vi "Import Export - Configuration Dialog.vi"(8 "error in":errorcluster, 11 "Item Ref in":T1 format="%.0x") -> (0 "error out":errorcluster, 3 "Item Ref out":T1 format="%.0x")   [LabVIEW 2017, in "PXImc System Explorer.lvlib"]
doc: "Goal of this VI is to prompt user to enter path t the configuration file and set Import or Export action over selected file.\n------------------------------------------------------------------------------------------------------\nIMPLEMENTATION\nCustom .net dialog window"
uses:
  PXImc System Explorer.lvlib
  <vilib>/NI Veristand/Custom Device API/Custom Device Item Ref.ctl
  <vilib>/event_ctls.llb/eventvkey.ctl
  Shared/Constants.vi
  <vilib>/NI Veristand/Custom Device API/Get Item Property (Path).vi
  <vilib>/NI Veristand/Custom Device API/Set Item Property (Path).vi
  <vilib>/NI VeriStand/Custom Device API/Custom Device API.lvlib
  Shared/PXImc Shared.lvlib
panel:
  in  "Forced?":bool=TRUE caption="Forced Import?"
  in  "dummy error cover":string
  in  "Import":bool
  in  "Close":bool
  in  "Export":bool
  in  "Configuration File Path":path
  # "File for Import/Export not found! Please seclect valid file to unlock this feature."
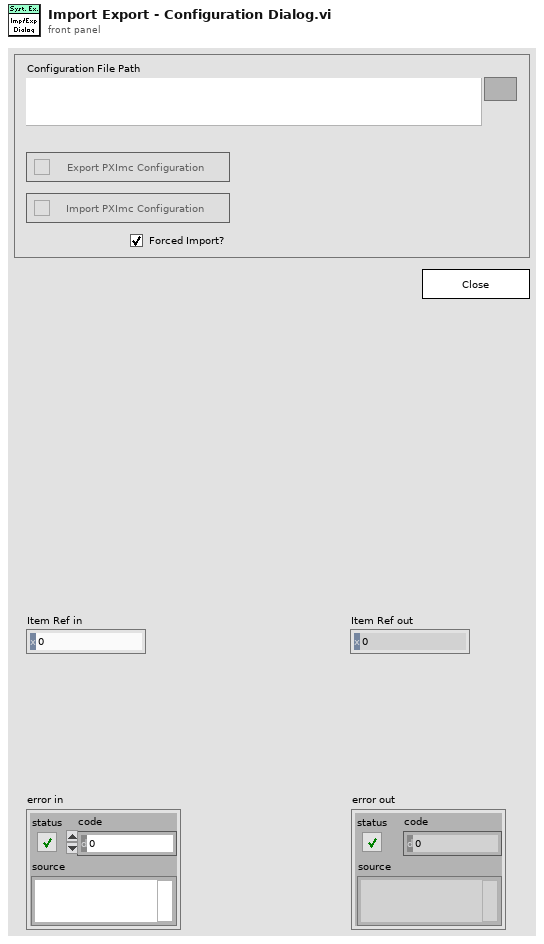
[diagram p1: front panel]
types:
  T1 = typedef "Custom Device API.lvlib/Custom Device Item Ref.ctl" = u64
  T2 = enum8{"Enabled", "Disabled", "Disabled and Grayed Out"}
  T3 = typedef "eventvkey.ctl" = enum16{"ASCII", "Enter", "Return", "Shift", "Ctrl", "Alt", "Cmd", "Opt", "Caps", "NumLock", "Clear", "Break", "Up", "Down", "Left", "Right", "Insert", "Delete", "Home", "End", "PageUp", "PageDown", "Escape", "Help", "Pause", "ScrollLock", "F1", "F2", "F3", "F4", "F5", "F6", "F7", "F8", "F9", "F10", "F11", "F12", "F13", "F14", "F15", "F16", "F17", "F18", "F19", "F20", "F21", "F22", "F23", "F24", "Play", "VolumeUp", "VolumeDown", "Mute", "Two Byte Char"}
  T4 = enum16{"open", "replace", "create", "open or create", "replace or create", "replace or create with confirmation"}
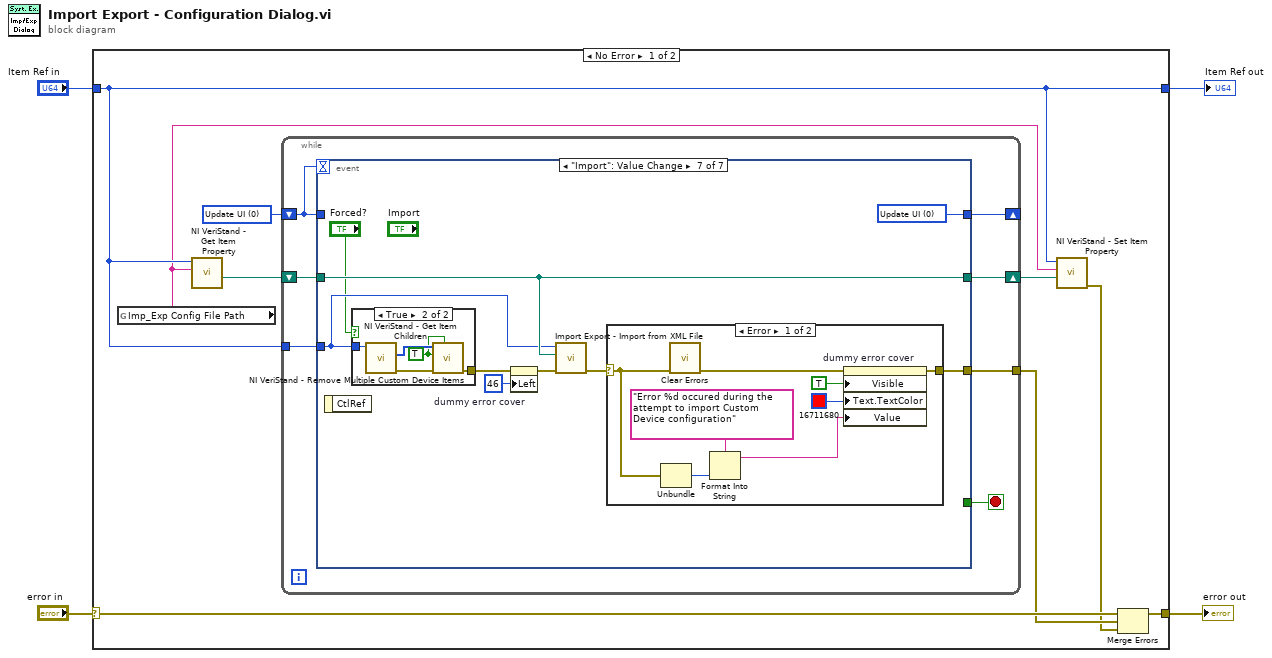
[diagram p0: block diagram]
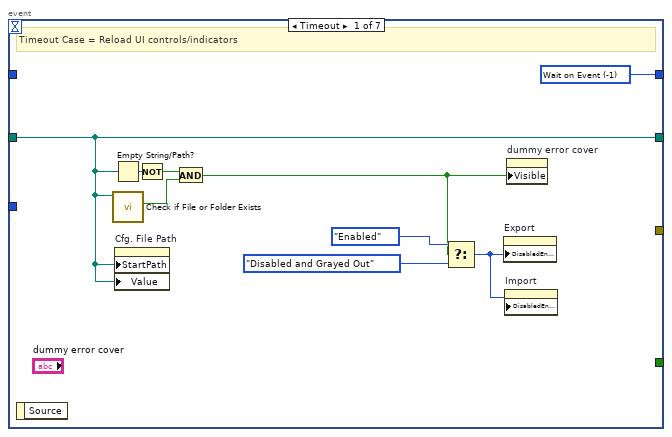
[diagram p2: hidden frame]
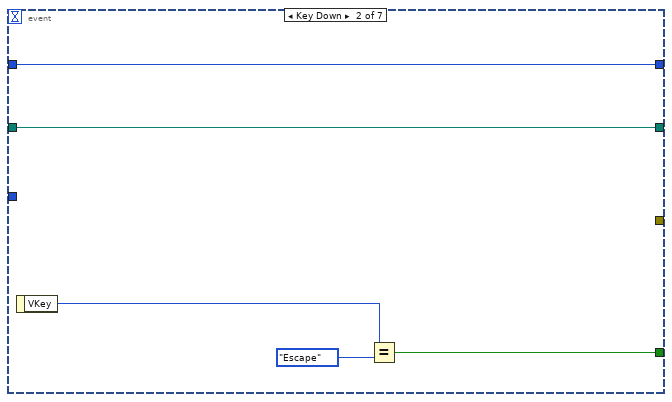
[diagram p3: hidden frame]
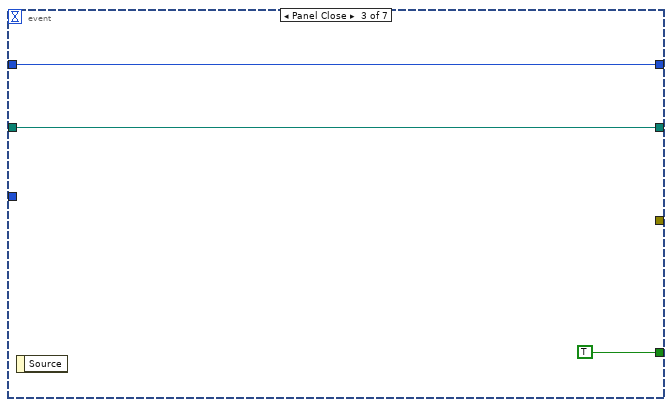
[diagram p4: hidden frame]
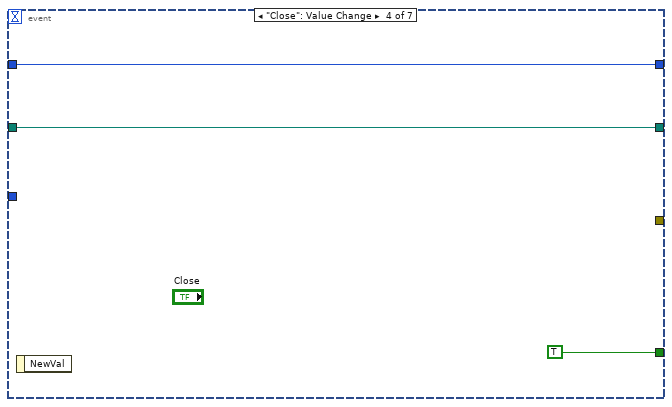
[diagram p5: hidden frame]
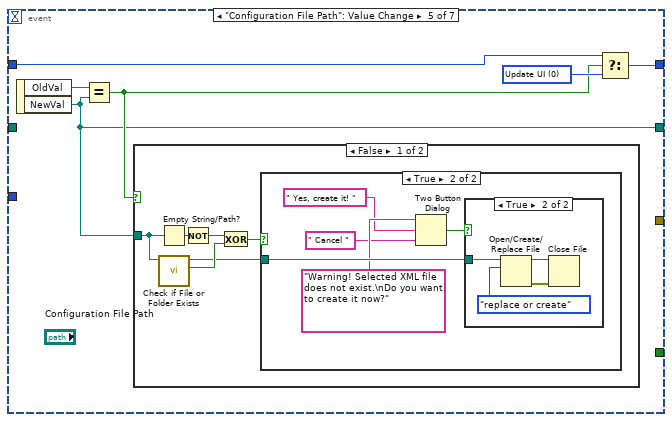
[diagram p6: hidden frame]
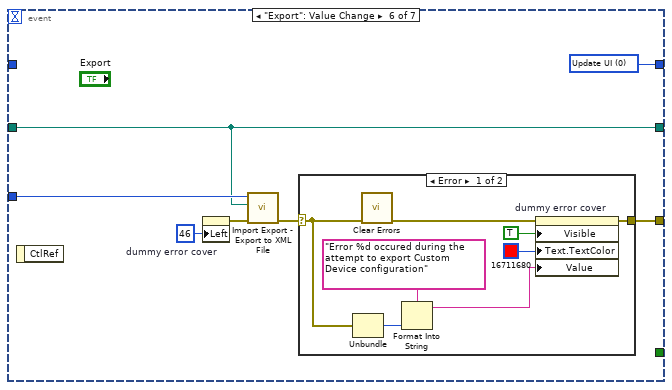
[diagram p10: hidden frame]
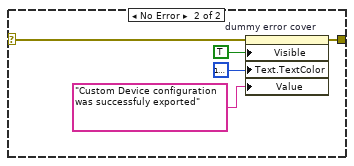
[diagram p11: hidden frame]
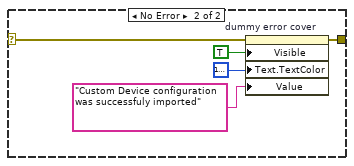
[diagram p13: hidden frame]
diagram:
  n1 = case shown="No Error" "error in" {
    selector: "error in" -> [w13 w109]
    tunnel: [w10 w109] -> w3
    tunnel: "Item Ref in" -> [w8 w110]
    tunnel: [w8 w110] -> w2
    frame No Error {
      w12 = 0 items=["Wait on Event"=-1, "Update UI"=0]
      n2 = global read "Constants.vi" "Imp_Exp Config File Path"() -> (w5:string)
      n3 = call-poly <vilib>:"NI VeriStand - Get Item Property.vi"("Property Name"=w5, "Item Ref in"=w8) -> ("Value"=w11:path)  [unwired: 6 in, 3 out]
      n4 = while {
        shift-right: [w19] -> _
        shift-left: w12 -> [w18]
        tunnel: w8 -> [w17]
        shift-right: [w16] -> w7
        shift-left: w11 -> [w15]
        tunnel: [w14] -> w9
        stop <- w20 stop-if-true
        n5 = event shown="[6] \"Import\": Value Change" {
          selector: _ -> [_ _ _ _ _ _ _]
          dyn-events: _ -> [_ _ _ _ _ _ _]
          timeout: w18 -> [_ _ _ _ _ _ _]
          tunnel: [_ w32 TRUE TRUE _ _ _] -> w20
          tunnel: [w29 w31 w37 w40 w43 w68 w90] -> w19
          tunnel: w18 -> [_ w31 w37 w40 w45 _ _]
          tunnel: w17 -> [_ _ _ _ _ w67 w83]
          tunnel: w15 -> [w28 w30 w36 w39 _ w66 w85]
          tunnel: [w28 w30 w36 w39 w41 w66 w85] -> w16
          tunnel: [_ _ _ _ _ w64 w88] -> w14
          event Timeout {
            w29 = -1 items=["Wait on Event"=-1, "Update UI"=0]
            # "Timeout Case = Reload UI controls/indicators"
            n6 = event-data() -> ()  [unwired: 1 in, 1 out]
            n7 = Empty String/Path?(string/path=w28) -> (empty?=w27:bool)
            n8 = call <vilib>:"Check if File or Folder Exists.vi"("path"=w28) -> ("file or folder exists?"=w26:bool)  [unwired: 8 in, 2 out]
            n9 = property on="Cfg. File Path" class="Path"("StartPath"=w28, "Value"=w28) -> ()  [unwired: 2 in, 2 out]
            n10 = Not(x=w27) -> (.not. x?=w25:bool)
            n11 = And(x=w25, y=w26) -> (x .and. y?=w22:bool)
            n12 = Select(t=T2."Enabled" ("Disabled"), s=w22, f=T2."Disabled and Grayed Out" ("Disabled")) -> (s? t:f=w23:T2)
            n13 = property on="Export" class="Bool"("DisabledEnum"=w23) -> ()  [unwired: 2 in, 2 out]
            n14 = property on="Import" class="Bool"("DisabledEnum"=w23) -> ()  [unwired: 2 in, 2 out]
            n15 = property on="dummy error cover" class="Str"("Visible"=w22) -> ()  [unwired: 2 in, 2 out]
          }
          event Key Down {
            n16 = event-data() -> ("VKey"=w33:T3)  [unwired: 1 in]
            n17 = Equal?(x=w33, y=eventvkey."Escape" ("VKey")) -> (x = y?=w32:bool)
          }
          event Panel Close {
            n18 = event-data() -> ()  [unwired: 1 in, 1 out]
          }
          event "Close": Value Change {
            n19 = event-data() -> ()  [unwired: 1 in, 1 out]
          }
          event "Configuration File Path": Value Change {
            w44 = 0 items=["Wait on Event"=-1, "Update UI"=0]
            n20 = event-data() -> ("OldVal"=w46:path, "NewVal"=w41:path)  [unwired: 1 in]
            n21 = Equal?(x=w46, y=w41) -> (x = y?=w42:bool)
            n22 = case shown="False" w42 {
              tunnel: w41 -> [w51 _]
              frame False {
                n23 = Empty String/Path?(string/path=w51) -> (empty?=w52:bool)
                n24 = call <vilib>:"Check if File or Folder Exists.vi"("path"=w51) -> ("file or folder exists?"=w50:bool, "dup path"=w47:path)  [unwired: 8 in, 1 out]
                n25 = Not(x=w52) -> (.not. x?=w49:bool)
                n26 = Exclusive Or(1:w50, 2:w49) -> (0:w48:bool)
                n27 = case shown="True" w48 {
                  tunnel: w47 -> [_ w57]
                  frame False {
                  }
                  frame True {
                    n28 = Two Button Dialog(message="Warning! Selected XML file does not exist.\nDo you want to create it now?", 1:" Cancel " ("F button name (\"Cancel\")"), 2:" Yes, create it! " ("T button name (\"OK\")")) -> (T button?=w56:bool)
                    n29 = case shown="True" w56 {
                      tunnel: w57 -> [_ w61]
                      frame False {
                      }
                      frame True {
                        n30 = Open/Create/Replace File(file path (use dialog)=w61, operation (0:open)=T4."replace or create") -> (refnum out=w59:refnum<file>, error out=w60:errorcluster)  [unwired: 4 in, 1 out]
                        n31 = Close File(refnum=w59, error in=w60) -> ()  [unwired: 2 out]
                      }
                    }
                  }
                }
              }
              frame True {
              }
            }
            n32 = Select(t=w45, s=w42, f=w44) -> (s? t:f=w43:i32)
          }
          event "Export": Value Change {
            w68 = 0 items=["Wait on Event"=-1, "Update UI"=0]
            n33 = event-data() -> ()  [unwired: 1 in, 1 out]
            n34 = property on="dummy error cover" class="Str"("Left"=46 ("Position:Left")) -> (error out=w63:errorcluster)  [unwired: 2 in, 1 out]
            n35 = call "Import Export - Export to XML File.vi"("error in"=w63, "Configuration File Path"=w66, "Item Ref in"=w67) -> ("error out"=w65:errorcluster)  [unwired: 6 in, 2 out]
            n36 = case shown="Error" w65 {
              selector: w65 -> [w73 w79]
              tunnel: [w76 w81] -> w64
              frame Error {
                n37 = Unbundle(w73) -> ("code"=w70:i32)  [unwired: 2 out]
                n38 = call <vilib>:"Clear Errors.vi"("error in (no error)"=w73) -> ("error out"=w74:errorcluster)  [unwired: 5 in, 1 out]
                n39 = Format Into String(format string="Error %d occured during the attempt to export Custom Device configuration" ("dummy error cover"), w70) -> (resulting string=w72:string)  [unwired: 2 in, 1 out]
                n40 = property on="dummy error cover" class="Str"(error in=w74, "Visible"=TRUE, "Text.TextColor"=u32 16711680, "Value"=w72) -> (error out=w76:errorcluster)  [unwired: 1 in, 1 out]
              }
              frame No Error {
                n41 = property on="dummy error cover" class="Str"(error in=w79, "Visible"=TRUE, "Text.TextColor"=u32 16777222, "Value"="Custom Device configuration was successfuly exported" ("dummy error cover")) -> (error out=w81:errorcluster)  [unwired: 1 in, 1 out]
              }
            }
          }
          event "Import": Value Change {
            w90 = 0 items=["Wait on Event"=-1, "Update UI"=0]
            n42 = event-data() -> ()  [unwired: 1 in, 1 out]
            n43 = case shown="True" "Forced?" {
              tunnel: w83 -> [_ w92]
              tunnel: [_ w91] -> w84
              frame False {
              }
              frame True {
                w93 = TRUE ("Force Delete (F)")
                n44 = call <vilib>:"NI VeriStand - Get Item Children.vi"("Item Ref in"=w92) -> ("error out"=w94:errorcluster, "Child Refs"=w95:T1[])  [unwired: 7 in, 2 out]
                n45 = call <vilib>:"NI VeriStand - Remove Multiple Custom Device Items.vi"("Skip action VI on delete (F)"=w93, "error in (no error)"=w94, "Force Delete (F)"=w93, "Item Refs in"=w95) -> ("error out"=w91:errorcluster)  [unwired: 6 in, 1 out]
              }
            }
            n46 = property on="dummy error cover" class="Str"(error in=w84, "Left"=46 ("Position:Left")) -> (error out=w86:errorcluster)  [unwired: 1 in, 1 out]
            n47 = call "Import Export - Import from XML File.vi"("error in"=w86, "Configuration File Path"=w85, "Item Ref in"=w83) -> ("error out"=w89:errorcluster)  [unwired: 6 in, 2 out]
            n48 = case shown="Error" w89 {
              selector: w89 -> [w100 w106]
              tunnel: [w103 w108] -> w88
              frame Error {
                n49 = Unbundle(w100) -> ("code"=w97:i32)  [unwired: 2 out]
                n50 = call <vilib>:"Clear Errors.vi"("error in (no error)"=w100) -> ("error out"=w101:errorcluster)  [unwired: 5 in, 1 out]
                n51 = Format Into String(format string="Error %d occured during the attempt to import Custom Device configuration" ("dummy error cover"), w97) -> (resulting string=w99:string)  [unwired: 2 in, 1 out]
                n52 = property on="dummy error cover" class="Str"(error in=w101, "Visible"=TRUE, "Text.TextColor"=u32 16711680, "Value"=w99) -> (error out=w103:errorcluster)  [unwired: 1 in, 1 out]
              }
              frame No Error {
                n53 = property on="dummy error cover" class="Str"(error in=w106, "Visible"=TRUE, "Text.TextColor"=u32 16777222, "Value"="Custom Device configuration was successfuly imported" ("dummy error cover")) -> (error out=w108:errorcluster)  [unwired: 1 in, 1 out]
              }
            }
          }
        }
      }
      n54 = call-poly <vilib>:"NI VeriStand - Set Item Property.vi"("Value"=w7, "Property Name"=w5, "Item Ref in"=w8) -> ("error out"=w6:errorcluster)  [unwired: 6 in, 2 out]
      n55 = Merge Errors(w13, w9, w6) -> (w10:errorcluster)
    }
    frame Error {
    }
  }
  "error out" <- w3
  "Item Ref out" <- w2
